vi "get_context.vi"(8 "error in (no error)":errorcluster, 11 "Queue Log Provider in":refnum<class "NIErrLog Log Provider.lvclass">) -> (0 "error out":errorcluster, 1 "context":string, 3 "Queue Log Provider out":refnum<class "NIErrLog Log Provider.lvclass">)   [LabVIEW 2019, in "LVCOOOP.lvlib" / "Utility API.lvlib" / "NIErrLog Log Provider.lvclass"]
uses:
  NIErrLog Log Provider.lvclass
  NIErrLog Log Provider.lvclass/NIErrLog Log Provider.ctl
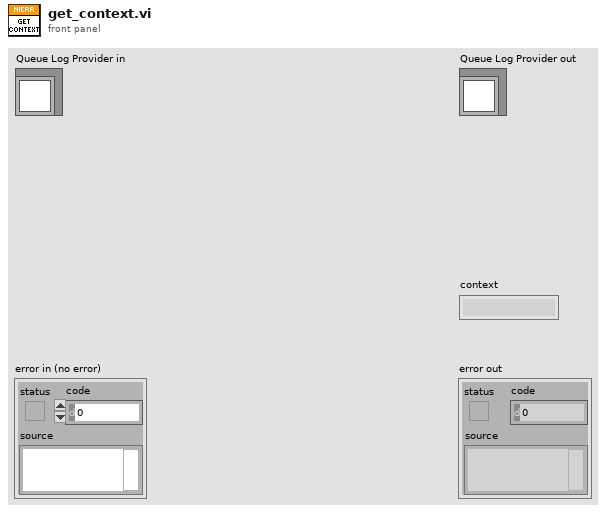
[diagram p1: front panel]
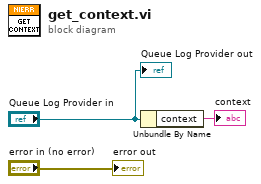
[diagram p0: block diagram]
diagram:
  n1 = Unbundle By Name("Queue Log Provider in") -> ("context"=→"context":string)
  "error out" <- "error in (no error)"
  "Queue Log Provider out" <- "Queue Log Provider in"
